vi "Image2ObjectsDistances.vi"(3 "error in (no error)":errorcluster, 5 "Image Src":T1) -> (0 "error out":errorcluster, 2 "Objects bottom cords":cluster{"Cord":cluster{"X":dbl, "Y":dbl}[]}[](array[cluster]))   [LabVIEW 2009, in "ImageAnalysis.lvlib"]
uses:
  ImageAnalysis.lvlib
  <vilib>/vision/Image Controls.llb/IMAQ Image.ctl
  ImageProcessing.lvlib
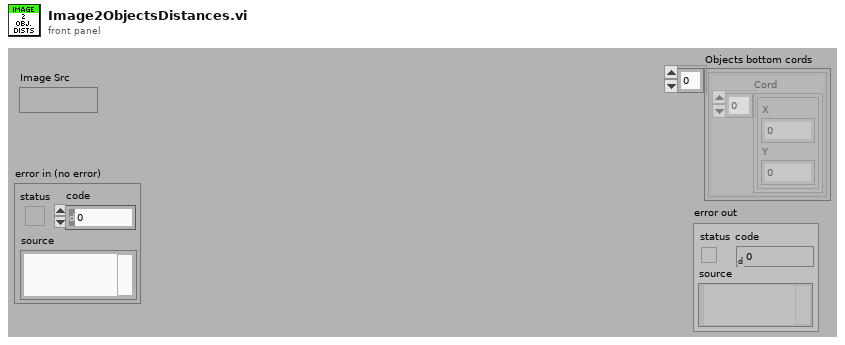
[diagram p1: front panel]
types:
  T1 = typedef "IMAQ Image.ctl" = refnum<image>
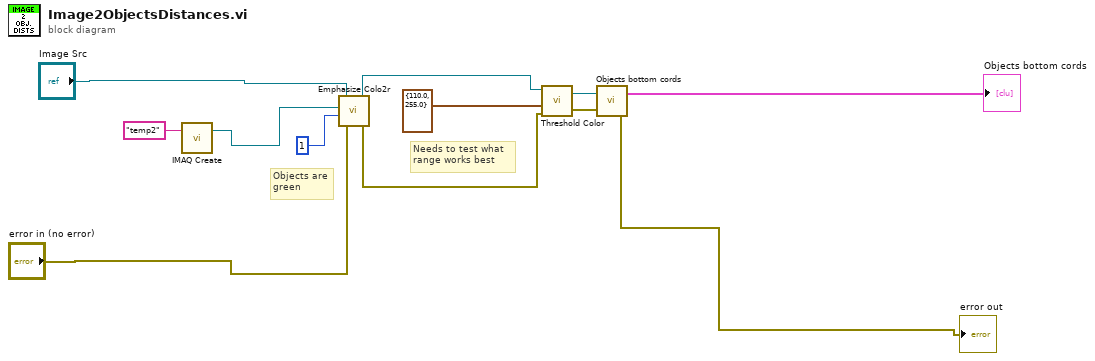
[diagram p0: block diagram]
diagram:
  # "Needs to test what \nrange works best"
  # "Objects are\ngreen"
  n1 = call "IMAQ Create"("Image Name"="temp2") -> ("New Image"=w1:T1)  [unwired: 4 in, 1 out]
  n2 = call "Emphasize Colo2r.vi"("error in (no error)"="error in (no error)", "Color"=i8 1, "Image Dst"=w1, "Image Src"="Image Src") -> ("error out"=w7:errorcluster, "Image Out"=w10:T1)
  n3 = call "Threshold Color.vi"("error in (no error)"=w7, "Range"=cluster{"Lower value":sgl, "Upper value":sgl} {"Lower value"=110.0, "Upper value"=255.0}, "Image Src"=w10) -> ("error out"=w4:errorcluster, "Image Dst Out"=w3:T1)  [unwired: 1 in]
  n4 = call "Objects bottom cords.vi"("error in (no error)"=w4, "Image"=w3) -> ("error out"=→"error out":errorcluster, "Objects bottom cords"=→"Objects bottom cords":cluster{"Cord":cluster{"X":dbl, "Y":dbl}[]}[])
